vi "Obtain Queue.vi"(8 "Error In":errorcluster, 11 "Name":string) -> (0 "Error Out":errorcluster, 3 "queue out":refnum<queue>)   [LabVIEW 2019, in "Queue.lvlib"]
uses:
  Queue.lvlib
  Message Cluster.ctl
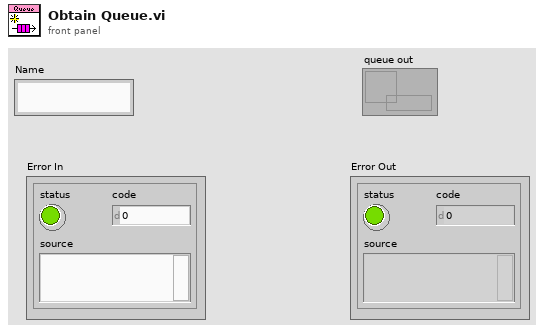
[diagram p1: front panel]
types:
  T1 = typedef "Queue.lvlib/Message Cluster.ctl" = cluster{"Message":string, "Data":variant}
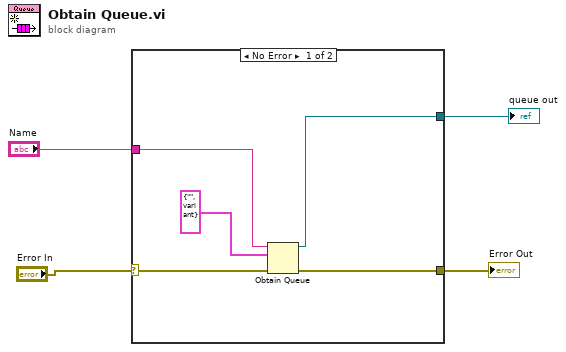
[diagram p0: block diagram]
diagram:
  n1 = case shown="No Error" "Error In" {
    selector: "Error In" -> [w8 w10]
    tunnel: [w7 w10] -> w3
    tunnel: "Name" -> [w9 _]
    tunnel: [w5 _] -> w1
    frame No Error {
      n2 = Obtain Queue(name (unnamed)=w9, element data type=T1 {"Message"="", "Data"=variant} ("Message Cluster"), error in (no error)=w8) -> (queue out=w5:refnum<queue>, error out=w7:errorcluster)  [unwired: 2 in, 1 out]
    }
    frame Error {
    }
  }
  "Error Out" <- w3
  "queue out" <- w1
